vi "Tipo de señal.vi"(8 "error in (no error)":errorcluster, 10 "Tipo señal":enum16{""}(ring), 11 "Measurement gg in":refnum<class "Measurement gg.lvclass">) -> (0 "error out":errorcluster, 3 "Measurement gg out":refnum<class "Measurement gg.lvclass">)   [LabVIEW 2020, in "Measurement gg.lvlib" / "Measurement gg.lvclass"]
uses:
  Measurement gg.lvclass
  Measurement gg.lvclass/Measurement gg.ctl
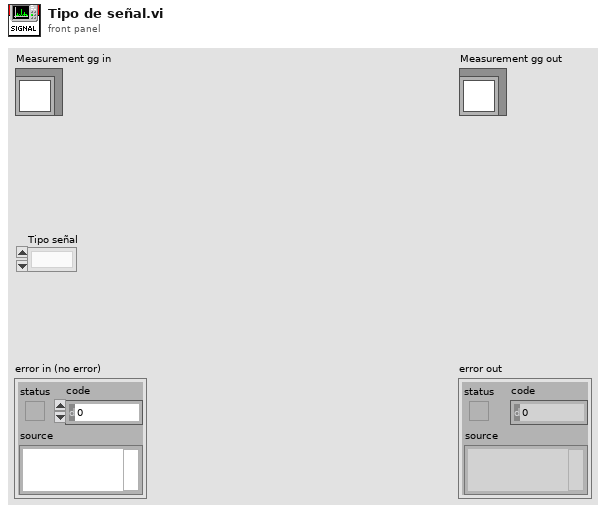
[diagram p1: front panel]
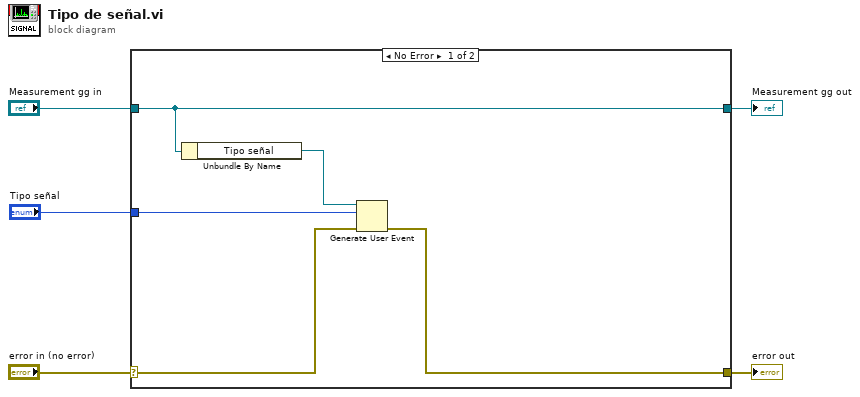
[diagram p0: block diagram]
diagram:
  n1 = case shown="No Error" "error in (no error)" {
    selector: "error in (no error)" -> [w9 w12]
    tunnel: [w8 w12] -> w4
    tunnel: [w7 w11] -> w2
    tunnel: "Measurement gg in" -> [w7 w11]
    tunnel: "Tipo señal" -> [w10 _]
    frame No Error {
      n2 = Unbundle By Name(w7) -> ("Tipo señal"=w6:refnum<user-event>)
      n3 = Generate User Event(user event=w6, event data cluster=w10, error in=w9) -> (error out=w8:errorcluster)  [unwired: 1 in, 1 out]
    }
    frame Error {
    }
  }
  "error out" <- w4
  "Measurement gg out" <- w2
